vi "BioFeedback21(v_0.2).vi"() -> ()   [LabVIEW 2016]
doc: "Use this template to build a producer/consumer design pattern. Use this template when you need to execute a process, such as data analysis, when a data source, such as a triggered acquisition, produces data at an uneven rate and you need to execute the process when the data becomes available."
uses:
  customSubVIs/8ChanWfmArray.ctl
  <vilib>/Utility/file.llb/Write Delimited Spreadsheet (string).vi
panel:
  in  "MVC Delay (s)":dbl=1.0
  out "trial last time":timestamp
  out "mvc last time":timestamp
  in  "Display Width for MVC (s)":dbl(slide) scale=0.1..10.0
  in  "Display Width for Current Trial":dbl(slide) scale=0.1..10.0
  out "Current Trial (Filtered)":waveform(dbl)(graph)
  out "Current MVC (Filtered)":waveform(dbl)(graph)
  in  "enableSave":bool caption="No Save      Save"
  in  "barOrGraph":bool=TRUE caption="Graph (under construction)       Bar"
  in  "Trial comment":string
  out "Collecting Data":bool
  in  "Display Min":dbl
  in  "Display Max":dbl=100.0
  in  "log filepath":path
  out "TrialStartTime":timestamp
  in  "Trial Duration (s)":dbl=3.0
  out "Trial Number":dbl
  in  "Session Name":string="Test"
  out "loopTime":dbl=30.0 caption="Upper Cut-Off"
  in  "trial display data":path
  out "Disp Data":cluster{"queue out":refnum<queue>, dbl, dbl}[](array[cluster])
  in  "Target Percentage":dbl=10.0
  out "Current Activation":dbl
  out "DisplayBarActivation":dbl(slide) caption="Percent Activation" max=1.0 scale=0.0..100.0
  in  "EMG Channel To Display":dbl=1.0
  out "MVC Data":cluster{"queue out":refnum<queue>, dbl, dbl}[](array[cluster])
  out "Trial Name":string="Test"
  in  "Data Directory":path=path "C:/Users/Tinggroup/Desktop/EMG Biofeedback System/LabviewFiles/Data"
  out "GetMaxStartTime":timestamp
  in  "MVC Number":dbl=1.0
  in  "MVC Duration (s)":dbl=3.0
  in  "Frames Per Second":dbl=30.0 caption="Upper Cut-Off"
  in  "EMG Input Device\nProduct Type":string="USB-6009"
  out "raw data":dynamicdata(graph)
  out "dispSize":dbl=20.0 caption="Lower Cut-Off"
  out "mvcSize":dbl=300.0 caption="Upper Cut-Off"
  in  "MVC Window Size (s)":dbl=0.5
  in  "Display Window Size (s)":dbl=0.5
  in  "MVC Raw Path":path
  in  "trial raw data":path
  in  "trial filtered data":path
  in  "MVC Filtered Path":path
  in  "Sample rate (Hz)":dbl=1000.0 caption="Upper Cut-Off"
  out "fps":dbl=20.0 caption="Lower Cut-Off"
  out "rate":dbl=300.0 caption="Upper Cut-Off"
  in  "Set Parameters":bool
  out "lower":dbl=20.0 caption="Lower Cut-Off"
  out "upper":dbl=300.0 caption="Upper Cut-Off"
  in  "Lower Cut-Off":dbl=20.0
  in  "Upper Cut-Off":dbl=500.0
  in  "Mark":bool
  in  "End Trial":bool
  in  "Get MVC":bool
  in  "StartTrial":bool
  out "State":T1(ring)
  out "FilteredAndRectified":waveform(dbl)[](graph) caption="Filtered and Rectified"
  in  "stop":bool
  # "Filtering"
  # "Add trial name\nBEFORE beginning trial"
  # "Display Settings"
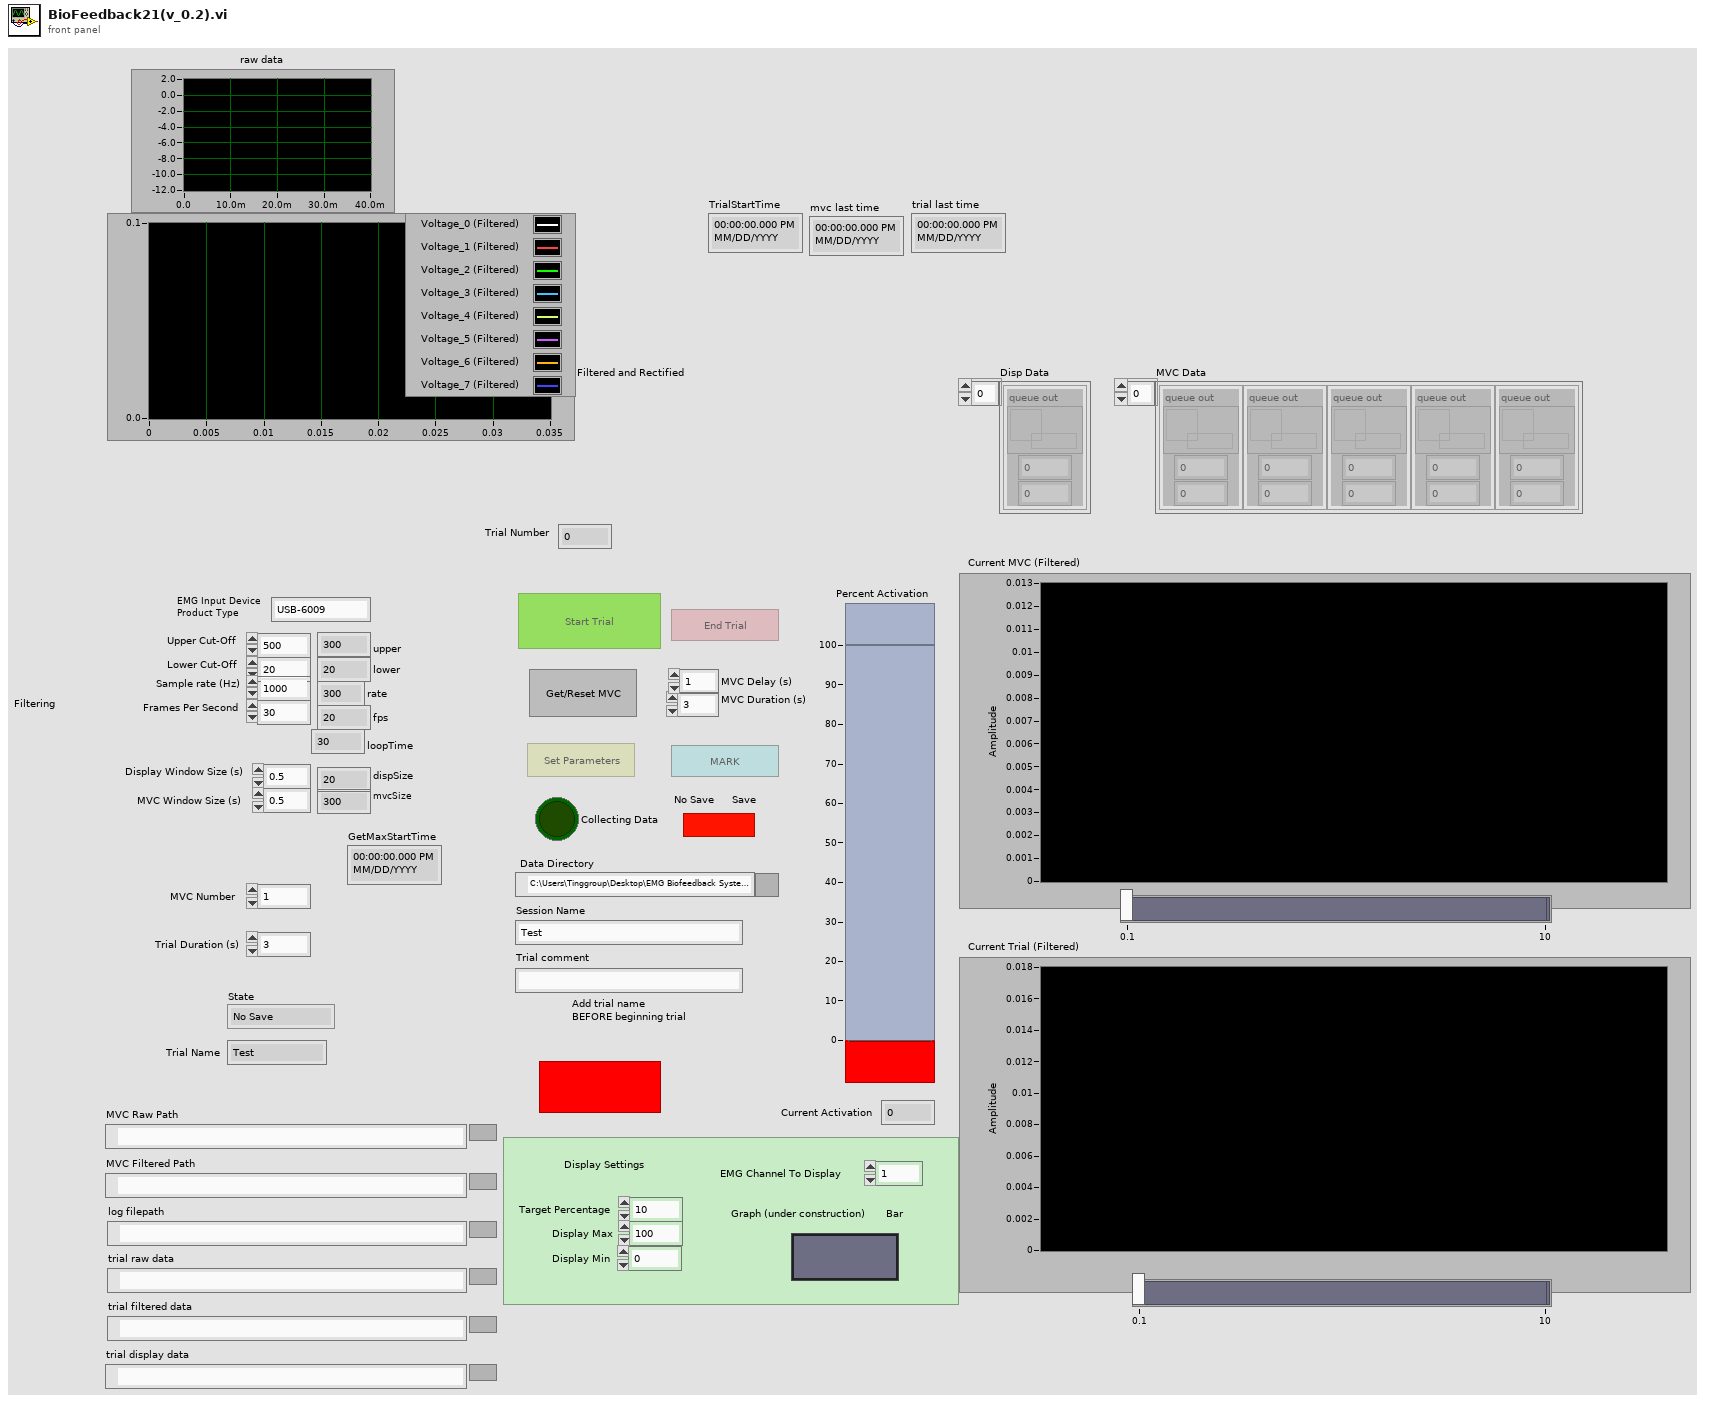
[diagram p1: front panel]
types:
  T1 = enum16{"No Save", "Acquiring Max", "Trial In Progress"}
  T2 = enum8{"Enabled", "Disabled", "Disabled and Grayed Out"}
  T3 = typedef "8ChanWfmArray.ctl" = waveform(dbl)[]
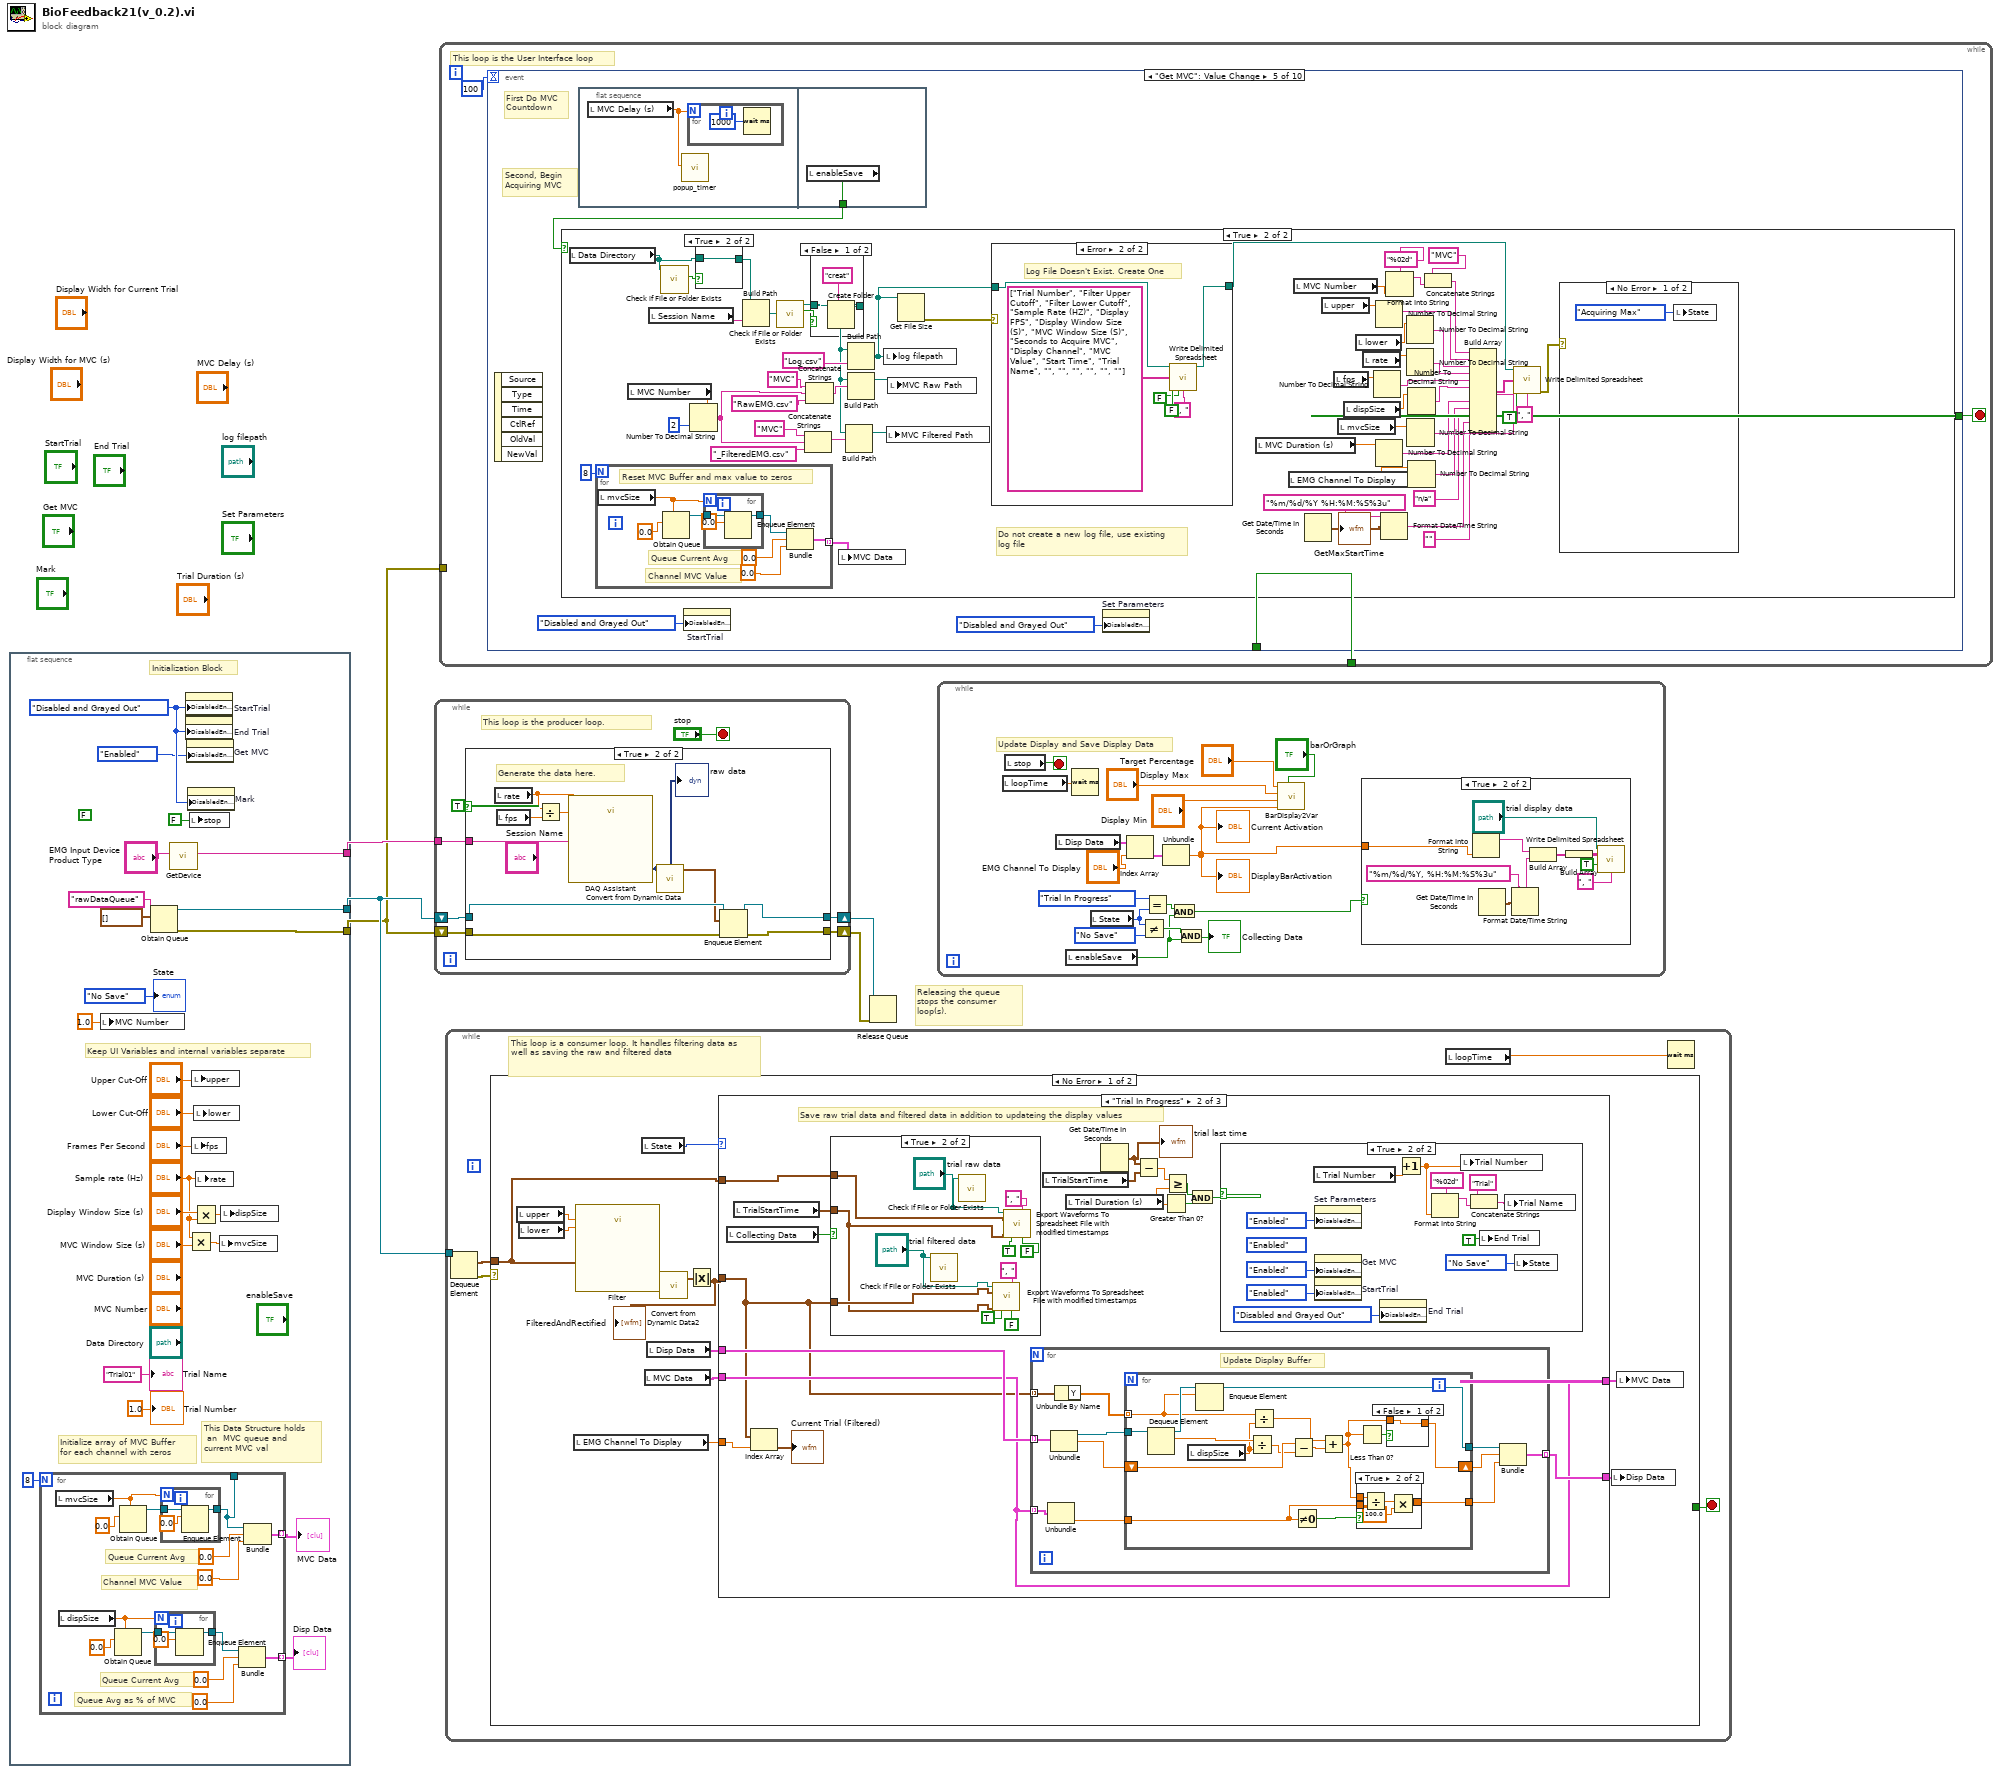
[diagram p0: block diagram]
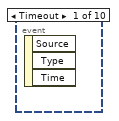
[diagram p3: hidden frame]
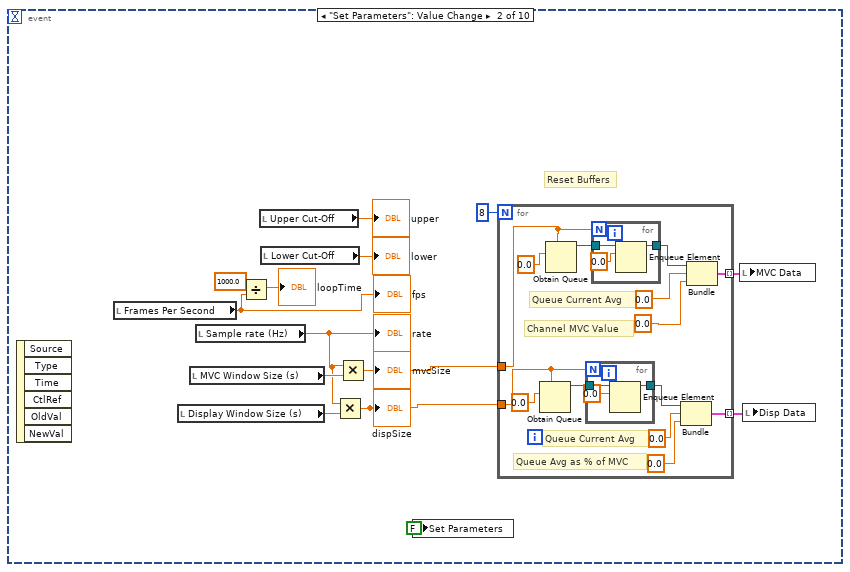
[diagram p4: hidden frame]
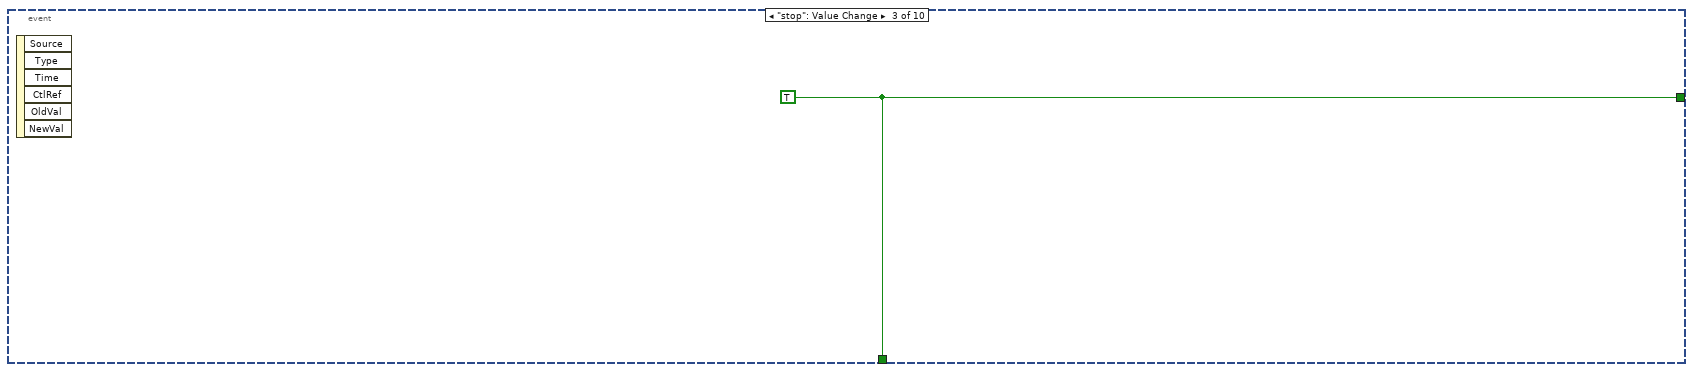
[diagram p5: hidden frame]
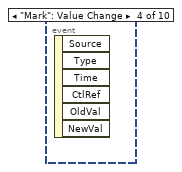
[diagram p6: hidden frame]
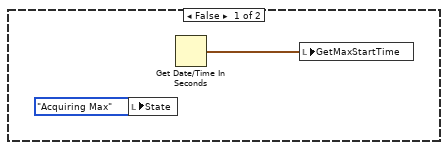
[diagram p7: hidden frame]
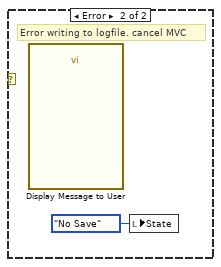
[diagram p8: hidden frame]
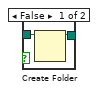
[diagram p11: hidden frame]
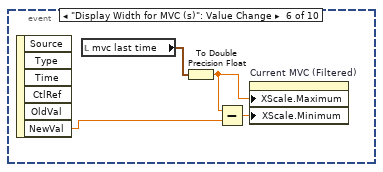
[diagram p12: hidden frame]
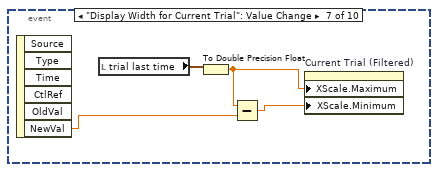
[diagram p13: hidden frame]
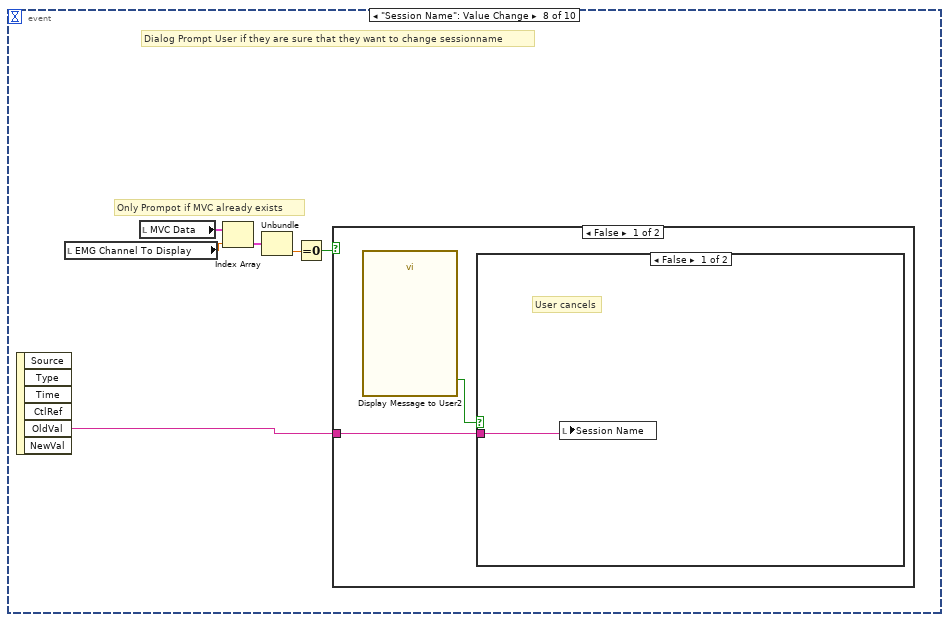
[diagram p14: hidden frame]
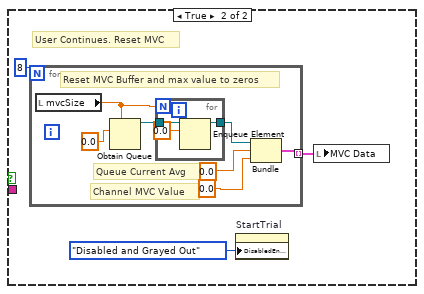
[diagram p15: hidden frame]
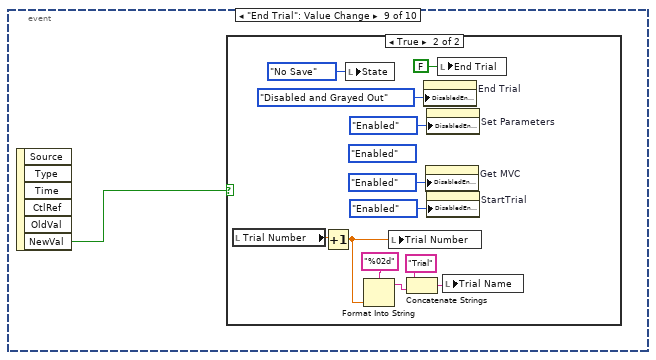
[diagram p17: hidden frame]
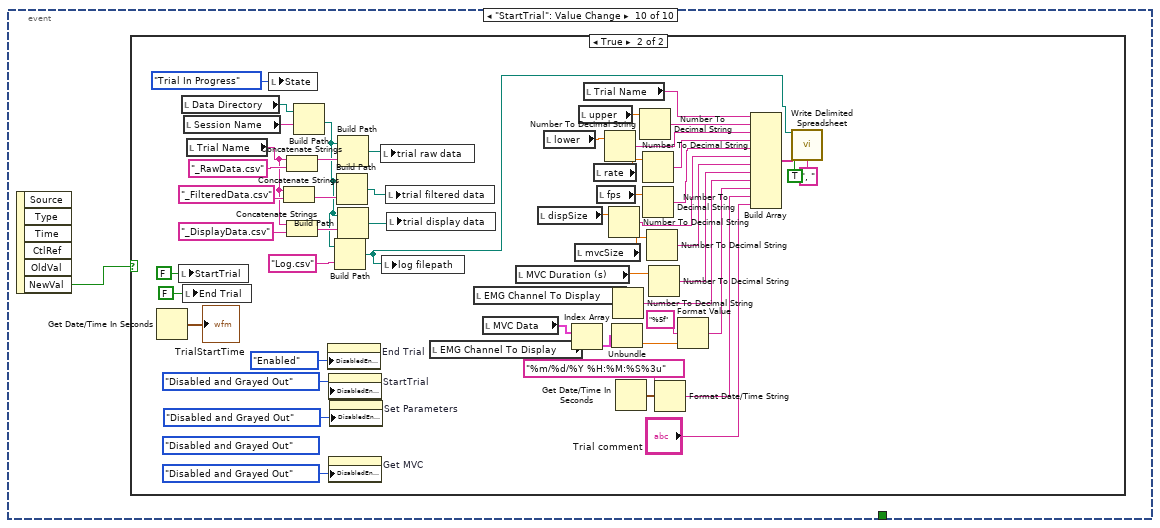
[diagram p19: hidden frame]
diagram:
  # "Releasing the queue stops the consumer loop(s)."
  n1 = flat-sequence {
    tunnel: [w20] -> w3
    tunnel: [w19] -> w2
    tunnel: [w22] -> w4
    frame #0 {
      (unwired) FALSE ("Visible")
      w27 = T2."Disabled and Grayed Out" ("Disabled")
      # "Keep UI Variables and internal variables separate"
      # "This Data Structure holds\n an  MVC queue and \ncurrent MVC val"
      # "Initialize array of MVC Buffer \nfor each channel with zeros"
      # "Initialization Block"
      n2 = for {
        N: 8 -> [_]
        tunnel: [w40] -> w12 mode=indexing
        tunnel: [w37] -> _
        tunnel: [w30] -> w11 mode=indexing
        # "Queue Avg as % of MVC"
        # "Queue Current Avg"
        # "Channel MVC Value"
        # "Queue Current Avg"
        n3 = local read "mvcSize"() -> (w41:dbl)
        n4 = local read "dispSize"() -> (w34:dbl)
        n5 = Obtain Queue(max queue size (-1, unlimited)=w34, element data type=0.0) -> (queue out=w31:refnum<queue>)  [unwired: 3 in, 2 out]
        n6 = Obtain Queue(max queue size (-1, unlimited)=w41, element data type=0.0) -> (queue out=w42:refnum<queue>)  [unwired: 3 in, 2 out]
        n7 = for {
          N: w34 -> [_]
          tunnel: w31 -> [w46]
          tunnel: [w44] -> w32
          n8 = Enqueue Element(queue=w46, element=0.0) -> (queue out=w44:refnum<queue>)  [unwired: 2 in, 2 out]
        }
        n9 = for {
          N: w41 -> [_]
          tunnel: w42 -> [w49]
          tunnel: [w47] -> w37
          n10 = Enqueue Element(queue=w49, element=0.0) -> (queue out=w47:refnum<queue>)  [unwired: 2 in, 2 out]
        }
        n11 = Bundle("queue out"=w32, 0.0, 0.0) -> (w30:cluster{"queue out":refnum<queue>, dbl, dbl})  [unwired: 1 in]
        n12 = Bundle("queue out"=w37, 0.0, 0.0) -> (w40:cluster{"queue out":refnum<queue>, dbl, dbl})  [unwired: 1 in]
      }
      "MVC Data" <- w12
      "Disp Data" <- w11
      n13 = local write "MVC Number"(1.0 ("MVC Number")) -> ()
      n14 = Obtain Queue(name (unnamed)="rawDataQueue", element data type=T3 [] ("initialized array")) -> (queue out=w20:refnum<queue>, error out=w19:errorcluster)  [unwired: 3 in, 1 out]
      n15 = call "GetDevice.vi"("EMG Input Device\nProduct Type"="EMG Input Device\nProduct Type") -> ("DAQmx Device Name"=w22:tag)  [unwired: 10 in]
      n16 = property on="StartTrial" class="Bool (strict)"("DisabledEnum"=w27) -> ()  [unwired: 2 in, 2 out]
      n17 = property on="End Trial" class="Bool (strict)"("DisabledEnum"=w27) -> ()  [unwired: 2 in, 2 out]
      n18 = property on="Get MVC" class="Bool"("DisabledEnum"=T2."Enabled" ("Disabled")) -> ()  [unwired: 2 in, 2 out]
      n19 = property on="Mark" class="Bool"("DisabledEnum"=w27) -> ()  [unwired: 2 in, 2 out]
      n20 = Multiply(x="Sample rate (Hz)", y="MVC Window Size (s)") -> (x*y=w14:dbl)
      n21 = local write "stop"(FALSE ("stop")) -> ()
      n22 = local write "upper"("Upper Cut-Off") -> ()
      n23 = local write "fps"("Frames Per Second") -> ()
      n24 = Multiply(x="Display Window Size (s)", y="Sample rate (Hz)") -> (x*y=w17:dbl)
      n25 = local write "lower"("Lower Cut-Off") -> ()
      n26 = local write "rate"("Sample rate (Hz)") -> ()
      n27 = local write "mvcSize"(w14) -> ()
      n28 = local write "dispSize"(w17) -> ()
      "Trial Name" <- "Trial01" ("Trial Name")
      "State" <- T1."No Save" ("State")
      "Trial Number" <- 1.0 ("Trial Number")
    }
  }
  n29 = while {
    shift-right: [w52] -> w1
    shift-left: w2 -> [w53]
    shift-right: [w54] -> w5
    shift-left: w3 -> [w55]
    tunnel: w4 -> [w50]
    stop <- "stop" stop-if-true
    # "This loop is the producer loop."
    n30 = case shown="True" TRUE ("Case Constant\n(See Context Help)") {
      tunnel: w55 -> [w58 w68]
      tunnel: [w58 w67] -> w54
      tunnel: w53 -> [w57 w66]
      tunnel: [w57 w65] -> w52
      tunnel: w50 -> [_ w60]
      frame False {
      }
      frame True {
        # "Generate the data here."
        n31 = local read "rate"() -> (w63:dbl)
        n32 = local read "fps"() -> (w64:dbl)
        n33 = Divide(x=w63, y=w64) -> (x/y=w62:dbl)
        n34 = call "DAQ Assistant"("rate"=w63, "number of samples"=w62, "device name"=w60) -> ("data"=w61:dynamicdata)  [unwired: 13 in, 3 out]
        "raw data" <- w61
        n35 = call "Convert from Dynamic Data"("Dynamic Data Type"=w61) -> ("Array of Waveform"=w59:waveform(dbl)[])  [unwired: 3 in]
        n36 = Enqueue Element(queue=w68, element=w59, error in (no error)=w66) -> (queue out=w67:refnum<queue>, error out=w65:errorcluster)  [unwired: 1 in, 1 out]
      }
    }
  }
  n37 = while {
    tunnel: [w71] -> _
    tunnel: w2 -> [_]
    stop <- w69 stop-if-true
    # "This loop is the User Interface loop"
    n38 = event shown="[4] \"Get MVC\": Value Change" {
      selector: _ -> [_ _ _ _ _ _ _ _ _ _]
      dyn-events: _ -> [_ _ _ _ _ _ _ _ _ _]
      timeout: u32 100 ("milliseconds to wait") -> [_ _ _ _ _ _ _ _ _ _]
      tunnel: [_ _ w106 _ _ _ _ _ _ _] -> w69
      tunnel: [_ _ w106 _ _ _ _ _ _ _] -> w71
      event Timeout {
        n39 = event-data() -> ()  [unwired: 1 in, 3 out]
      }
      event "Set Parameters": Value Change {
        # "Reset Buffers"
        n40 = event-data() -> ()  [unwired: 1 in, 6 out]
        n41 = local read "Frames Per Second"() -> (w73:dbl)
        "fps" <- w73
        n42 = local read "Display Window Size (s)"() -> (w83:dbl)
        n43 = local read "MVC Window Size (s)"() -> (w84:dbl)
        n44 = local read "Sample rate (Hz)"() -> (w81:dbl)
        "rate" <- w81
        n45 = Divide(x=1000.0, y=w73) -> (x/y=→"loopTime":dbl)
        n46 = local read "Upper Cut-Off"() -> (→"upper":dbl)
        n47 = local read "Lower Cut-Off"() -> (→"lower":dbl)
        n48 = Multiply(x=w81, y=w83) -> (x*y=w79:dbl)
        "dispSize" <- w79
        n49 = Multiply(x=w81, y=w84) -> (x*y=w80:dbl)
        "mvcSize" <- w80
        n50 = local write "Set Parameters"(FALSE ("Set Parameters")) -> ()
        n51 = for {
          N: 8 -> [_]
          tunnel: [w97] -> w77 mode=indexing
          tunnel: [w88] -> w78 mode=indexing
          tunnel: w80 -> [w87]
          tunnel: w79 -> [w86]
          # "Queue Avg as % of MVC"
          # "Queue Current Avg"
          # "Channel MVC Value"
          # "Queue Current Avg"
          n52 = Obtain Queue(max queue size (-1, unlimited)=w86, element data type=0.0) -> (queue out=w89:refnum<queue>)  [unwired: 3 in, 2 out]
          n53 = Obtain Queue(max queue size (-1, unlimited)=w87, element data type=0.0) -> (queue out=w98:refnum<queue>)  [unwired: 3 in, 2 out]
          n54 = for {
            N: w86 -> [_]
            tunnel: w89 -> [w102]
            tunnel: [w100] -> w90
            n55 = Enqueue Element(queue=w102, element=0.0) -> (queue out=w100:refnum<queue>)  [unwired: 2 in, 2 out]
          }
          n56 = for {
            N: w87 -> [_]
            tunnel: w98 -> [w105]
            tunnel: [w103] -> w94
            n57 = Enqueue Element(queue=w105, element=0.0) -> (queue out=w103:refnum<queue>)  [unwired: 2 in, 2 out]
          }
          n58 = Bundle("queue out"=w90, 0.0, 0.0) -> (w88:cluster{"queue out":refnum<queue>, dbl, dbl})  [unwired: 1 in]
          n59 = Bundle("queue out"=w94, 0.0, 0.0) -> (w97:cluster{"queue out":refnum<queue>, dbl, dbl})  [unwired: 1 in]
        }
        n60 = local write "MVC Data"(w77) -> ()
        n61 = local write "Disp Data"(w78) -> ()
      }
      event "stop": Value Change {
        w106 = TRUE
        n62 = event-data() -> ()  [unwired: 1 in, 6 out]
      }
      event "Mark": Value Change {
        n63 = event-data() -> ()  [unwired: 1 in, 6 out]
      }
      event "Get MVC": Value Change {
        # "Second, Begin \nAcquiring MVC"
        # "First Do MVC\nCountdown"
        n64 = event-data() -> ()  [unwired: 1 in, 6 out]
        n65 = case shown="True" w107 {
          frame False {
            n66 = local write "State"(T1."Acquiring Max" ("State")) -> ()
            n67 = Get Date/Time In Seconds() -> (seconds since 1Jan1904=w113:timestamp)
            n68 = local write "GetMaxStartTime"(w113) -> ()
          }
          frame True {
            # "Do not create a new log file, use existing \nlog file"
            n69 = local read "Data Directory"() -> (w122:path)
            n70 = for {
              N: 8 -> [_]
              tunnel: [w172] -> w119 mode=indexing
              # "Channel MVC Value"
              # "Queue Current Avg"
              # "Reset MVC Buffer and max value to zeros"
              n71 = local read "mvcSize"() -> (w175:dbl)
              n72 = Obtain Queue(max queue size (-1, unlimited)=w175, element data type=0.0) -> (queue out=w174:refnum<queue>)  [unwired: 3 in, 2 out]
              n73 = for {
                N: w175 -> [_]
                tunnel: w174 -> [w181]
                tunnel: [w179] -> w176
                n74 = Enqueue Element(queue=w181, element=0.0) -> (queue out=w179:refnum<queue>)  [unwired: 2 in, 2 out]
              }
              n75 = Bundle("queue out"=w176, 0.0, 0.0) -> (w172:cluster{"queue out":refnum<queue>, dbl, dbl})  [unwired: 1 in]
            }
            n76 = local read "MVC Number"() -> (w163:dbl)
            n77 = local read "Session Name"() -> (w162:string)
            n78 = call <vilib>:"Check if File or Folder Exists.vi"("path"=w122) -> ("file or folder exists?"=w123:bool)  [unwired: 8 in, 2 out]
            n79 = Number To Decimal String(number=w163, width (-)=i16 2) -> (decimal integer string=w144:string)
            n80 = case shown="True" w123 {
              tunnel: [w194 w195] -> w158
              tunnel: w122 -> [w193 w195]
              frame False {
                n81 = Create Folder(path (use dialog)=w193) -> (created path=w194:path)  [unwired: 2 in, 2 out]
              }
              frame True {
              }
            }
            n82 = Build Path(base path=w158, name or relative path=w162) -> (appended path=w161:path)
            n83 = call <vilib>:"Check if File or Folder Exists.vi"("path"=w161) -> ("file or folder exists?"=w160:bool, "dup path"=w159:path)  [unwired: 8 in, 1 out]
            n84 = Concatenate Strings("MVC" ("string"), w144, "_FilteredEMG.csv" ("string")) -> (w168:string)
            n85 = Concatenate Strings("MVC" ("string"), w144, "RawEMG.csv" ("string")) -> (w167:string)
            n86 = case shown="False" w160 {
              tunnel: w159 -> [w191 w192]
              tunnel: [w190 w192] -> w155
              frame False {
                n87 = Create Folder(prompt (Create Folder)="creat", path (use dialog)=w191) -> (created path=w190:path)  [unwired: 1 in, 2 out]
              }
              frame True {
              }
            }
            n88 = local write "MVC Data"(w119) -> ()
            n89 = Build Path(base path=w155, name or relative path=w168) -> (appended path=w120:path)
            n90 = Build Path(base path=w155, name or relative path="Log.csv" ("string")) -> (appended path=w116:path)
            n91 = Build Path(base path=w155, name or relative path=w167) -> (appended path=w121:path)
            n92 = local write "log filepath"(w116) -> ()
            n93 = local write "MVC Filtered Path"(w120) -> ()
            n94 = local write "MVC Raw Path"(w121) -> ()
            n95 = Get File Size(file=w116) -> (0:w115:errorcluster)  [unwired: 1 in, 2 out]
            n96 = case shown="Error" w115 {
              tunnel: [w182 w184] -> w135
              tunnel: w116 -> [w182 w183]
              frame No Error {
              }
              frame Error {
                # "Log File Doesn't Exist. Create One"
                n97 = call-poly <vilib>:"Write Delimited Spreadsheet.vi"("file path (dialog if empty)"=w183, "1D data"=string[] ["Trial Number", "Filter Upper Cutoff", "Filter Lower Cutoff", "Sample Rate (HZ)", "Display FPS", "Display Window Size (S)", "MVC Window Size (S)", "Seconds to Acquire MVC", "Display Channel", "MVC Value", "Start Time", "Trial Name", "", "", "", "", "", ""], "append to file? (new file:F)"=FALSE, "transpose? (no:F)"=FALSE, "delimiter (\\t)"=", " ("delimiter (\\t)")) -> ("new file path (Not A Path if cancelled)"=w184:path)  [unwired: 9 in, 1 out]
              }
            }
            n98 = local read "MVC Duration (s)"() -> (w149:dbl)
            n99 = local read "EMG Channel To Display"() -> (w148:dbl)
            n100 = local read "MVC Number"() -> (w131:dbl)
            n101 = Get Date/Time In Seconds() -> (seconds since 1Jan1904=w127:timestamp)
            "GetMaxStartTime" <- w127
            n102 = local read "upper"() -> (w154:dbl)
            n103 = local read "fps"() -> (w151:dbl)
            n104 = local read "mvcSize"() -> (w150:dbl)
            n105 = local read "dispSize"() -> (w145:dbl)
            n106 = local read "lower"() -> (w153:dbl)
            n107 = local read "rate"() -> (w152:dbl)
            n108 = Number To Decimal String(number=w151) -> (decimal integer string=w141:string)  [unwired: 1 in]
            n109 = Number To Decimal String(number=w154) -> (decimal integer string=w129:string)  [unwired: 1 in]
            n110 = Number To Decimal String(number=w149) -> (decimal integer string=w138:string)  [unwired: 1 in]
            n111 = Format Date/Time String(time format string (%c)="%m/%d/%Y %H:%M:%S%3u", seconds (now)=w127) -> (date/time string=w125:string)  [unwired: 1 in]
            n112 = Format Into String(format string="%02d", w131) -> (resulting string=w134:string)  [unwired: 2 in, 1 out]
            n113 = Number To Decimal String(number=w153) -> (decimal integer string=w143:string)  [unwired: 1 in]
            n114 = Number To Decimal String(number=w152) -> (decimal integer string=w142:string)  [unwired: 1 in]
            n115 = Number To Decimal String(number=w150) -> (decimal integer string=w139:string)  [unwired: 1 in]
            n116 = Number To Decimal String(number=w145) -> (decimal integer string=w140:string)  [unwired: 1 in]
            n117 = Number To Decimal String(number=w148) -> (decimal integer string=w137:string)  [unwired: 1 in]
            n118 = Concatenate Strings("MVC" ("string"), w134) -> (w130:string)
            n119 = Build Array(w130, w129, w143, w142, w141, w140, w139, w138, w137, "n/a", w125, "" ("element")) -> (w147:string[])
            n120 = call-poly <vilib>:"Write Delimited Spreadsheet.vi"("file path (dialog if empty)"=w135, "1D data"=w147, "append to file? (new file:F)"=TRUE, "delimiter (\\t)"=", " ("delimiter (\\t)")) -> ("error out"=w117:errorcluster)  [unwired: 10 in, 1 out]
            n121 = case shown="No Error" w117 {
              frame No Error {
                n122 = local write "State"(T1."Acquiring Max" ("State")) -> ()
              }
              frame Error {
                # "Error writing to logfile. cancel MVC"
                n123 = call "Display Message to User"() -> ()  [unwired: 10 in, 2 out]
                n124 = local write "State"(T1."No Save" ("State")) -> ()
              }
            }
          }
        }
        n125 = flat-sequence {
          tunnel: [w112] -> w107
          frame #0 {
            n126 = local read "MVC Delay (s)"() -> (w110:dbl)
            n127 = call "popup_timer.vi"("Seconds"=w110) -> ()  [unwired: 9 in, 1 out]
            n128 = for {
              N: w110 -> [_]
              n129 = Wait (ms)(milliseconds to wait=u32 1000) -> ()  [unwired: 1 out]
            }
          }
          frame #1 {
            n130 = local read "enableSave"() -> (w112:bool)
          }
        }
        n131 = property on="StartTrial" class="Bool (strict)"("DisabledEnum"=T2."Disabled and Grayed Out" ("Disabled")) -> ()  [unwired: 2 in, 2 out]
        n132 = property on="Set Parameters" class="Bool (strict)"("DisabledEnum"=T2."Disabled and Grayed Out" ("Disabled")) -> ()  [unwired: 2 in, 2 out]
      }
      event "Display Width for MVC (s)": Value Change {
        n133 = event-data() -> ("NewVal"=w199:dbl)  [unwired: 1 in, 5 out]
        n134 = local read "mvc last time"() -> (w196:timestamp)
        n135 = To Double Precision Float(number=w196) -> (double precision float=w197:dbl)
        n136 = Subtract(x=w197, y=w199) -> (x-y=w198:dbl)
        n137 = property on="Current MVC (Filtered)" class="WFChart (strict)"("XScale.Maximum"=w197, "XScale.Minimum"=w198) -> ()  [unwired: 2 in, 2 out]
      }
      event "Display Width for Current Trial": Value Change {
        n138 = event-data() -> ("NewVal"=w202:dbl)  [unwired: 1 in, 5 out]
        n139 = local read "trial last time"() -> (w203:timestamp)
        n140 = To Double Precision Float(number=w203) -> (double precision float=w201:dbl)
        n141 = Subtract(x=w201, y=w202) -> (x-y=w200:dbl)
        n142 = property on="Current Trial (Filtered)" class="WFChart (strict)"("XScale.Maximum"=w201, "XScale.Minimum"=w200) -> ()  [unwired: 2 in, 2 out]
      }
      event "Session Name": Value Change {
        # "Only Prompot if MVC already exists"
        # "Dialog Prompt User if they are sure that they want to change sessionname"
        n143 = event-data() -> ("OldVal"=w204:string)  [unwired: 1 in, 5 out]
        n144 = local read "EMG Channel To Display"() -> (w208:dbl)
        n145 = local read "MVC Data"() -> (w209:cluster{"queue out":refnum<queue>, dbl, dbl}[])
        n146 = Index Array(array=w209, index=w208) -> (element=w207:cluster{"queue out":refnum<queue>, dbl, dbl})
        n147 = Unbundle(w207) -> (w206:dbl)  [unwired: 2 out]
        n148 = Equal To 0?(x=w206) -> (x = 0?=w205:bool)
        n149 = case shown="False" w205 {
          tunnel: w204 -> [w210 _]
          frame False {
            n150 = call "Display Message to User2"() -> ("Change"=w211:bool)  [unwired: 10 in, 1 out]
            n151 = case shown="False" w211 {
              tunnel: w210 -> [w212 _]
              frame False {
                # "User cancels"
                n152 = local write "Session Name"(w212) -> ()
              }
              frame True {
                # "User Continues. Reset MVC"
                n153 = for {
                  N: 8 -> [_]
                  tunnel: [w216] -> w215 mode=indexing
                  # "Channel MVC Value"
                  # "Queue Current Avg"
                  # "Reset MVC Buffer and max value to zeros"
                  n154 = local read "mvcSize"() -> (w219:dbl)
                  n155 = Obtain Queue(max queue size (-1, unlimited)=w219, element data type=0.0) -> (queue out=w218:refnum<queue>)  [unwired: 3 in, 2 out]
                  n156 = for {
                    N: w219 -> [_]
                    tunnel: w218 -> [w225]
                    tunnel: [w223] -> w220
                    n157 = Enqueue Element(queue=w225, element=0.0) -> (queue out=w223:refnum<queue>)  [unwired: 2 in, 2 out]
                  }
                  n158 = Bundle("queue out"=w220, 0.0, 0.0) -> (w216:cluster{"queue out":refnum<queue>, dbl, dbl})  [unwired: 1 in]
                }
                n159 = property on="StartTrial" class="Bool (strict)"("DisabledEnum"=T2."Disabled and Grayed Out" ("Disabled")) -> ()  [unwired: 2 in, 2 out]
                n160 = local write "MVC Data"(w215) -> ()
              }
            }
          }
          frame True {
          }
        }
      }
      event "End Trial": Value Change {
        n161 = event-data() -> ("NewVal"=w226:bool)  [unwired: 1 in, 5 out]
        n162 = case shown="True" w226 {
          frame False {
          }
          frame True {
            (unwired) T2."Enabled" ("Disabled")
            n163 = local read "Trial Number"() -> (w231:dbl)
            n164 = Increment(x=w231) -> (x+1=w227:dbl)
            n165 = local write "State"(T1."No Save" ("State")) -> ()
            n166 = Format Into String(format string="%02d", w227) -> (resulting string=w230:string)  [unwired: 2 in, 1 out]
            n167 = local write "Trial Number"(w227) -> ()
            n168 = Concatenate Strings("Trial" ("string"), w230) -> (w232:string)
            n169 = property on="End Trial" class="Bool (strict)"("DisabledEnum"=T2."Disabled and Grayed Out" ("Disabled")) -> ()  [unwired: 2 in, 2 out]
            n170 = property on="Get MVC" class="Bool"("DisabledEnum"=T2."Enabled" ("Disabled")) -> ()  [unwired: 2 in, 2 out]
            n171 = property on="Set Parameters" class="Bool (strict)"("DisabledEnum"=T2."Enabled" ("Disabled")) -> ()  [unwired: 2 in, 2 out]
            n172 = property on="StartTrial" class="Bool (strict)"("DisabledEnum"=T2."Enabled" ("Disabled")) -> ()  [unwired: 2 in, 2 out]
            n173 = local write "End Trial"(FALSE ("End Trial")) -> ()
            n174 = local write "Trial Name"(w232) -> ()
          }
        }
      }
      event "StartTrial": Value Change {
        n175 = event-data() -> ("NewVal"=w239:bool)  [unwired: 1 in, 5 out]
        n176 = case shown="True" w239 {
          frame False {
          }
          frame True {
            (unwired) T2."Disabled and Grayed Out" ("Disabled")
            n177 = Get Date/Time In Seconds() -> (seconds since 1Jan1904=→"TrialStartTime":timestamp)
            n178 = local write "StartTrial"(FALSE ("StartTrial")) -> ()
            n179 = local read "Data Directory"() -> (w284:path)
            n180 = local write "End Trial"(FALSE ("End Trial")) -> ()
            n181 = local read "Session Name"() -> (w283:string)
            n182 = local read "Trial Name"() -> (w267:string)
            n183 = local write "State"(T1."Trial In Progress" ("State")) -> ()
            n184 = Concatenate Strings(w267, "_FilteredData.csv" ("string")) -> (w288:string)
            n185 = Concatenate Strings(w267, "_RawData.csv" ("string")) -> (w286:string)
            n186 = Concatenate Strings(w267, "_DisplayData.csv" ("string")) -> (w290:string)
            n187 = Build Path(base path=w284, name or relative path=w283) -> (appended path=w266:path)
            n188 = property on="End Trial" class="Bool (strict)"("DisabledEnum"=T2."Enabled" ("Disabled")) -> ()  [unwired: 2 in, 2 out]
            n189 = property on="StartTrial" class="Bool (strict)"("DisabledEnum"=T2."Disabled and Grayed Out" ("Disabled")) -> ()  [unwired: 2 in, 2 out]
            n190 = property on="Get MVC" class="Bool"("DisabledEnum"=T2."Disabled and Grayed Out" ("Disabled")) -> ()  [unwired: 2 in, 2 out]
            n191 = property on="Set Parameters" class="Bool (strict)"("DisabledEnum"=T2."Disabled and Grayed Out" ("Disabled")) -> ()  [unwired: 2 in, 2 out]
            n192 = Build Path(base path=w266, name or relative path="Log.csv" ("string")) -> (appended path=w250:path)
            n193 = Build Path(base path=w266, name or relative path=w288) -> (appended path=w282:path)
            n194 = Build Path(base path=w266, name or relative path=w286) -> (appended path=w281:path)
            n195 = Build Path(base path=w266, name or relative path=w290) -> (appended path=w291:path)
            n196 = local write "trial raw data"(w281) -> ()
            n197 = local write "log filepath"(w250) -> ()
            n198 = local write "trial filtered data"(w282) -> ()
            n199 = local write "trial display data"(w291) -> ()
            n200 = local read "EMG Channel To Display"() -> (w246:dbl)
            n201 = local read "EMG Channel To Display"() -> (w276:dbl)
            n202 = local read "MVC Data"() -> (w247:cluster{"queue out":refnum<queue>, dbl, dbl}[])
            n203 = local read "MVC Duration (s)"() -> (w275:dbl)
            n204 = local read "dispSize"() -> (w273:dbl)
            n205 = local read "lower"() -> (w270:dbl)
            n206 = Index Array(array=w247, index=w246) -> (element=w245:cluster{"queue out":refnum<queue>, dbl, dbl})
            n207 = local read "mvcSize"() -> (w274:dbl)
            n208 = local read "upper"() -> (w269:dbl)
            n209 = local read "Trial Name"() -> (w263:string)
            n210 = local read "rate"() -> (w271:dbl)
            n211 = local read "fps"() -> (w272:dbl)
            n212 = Number To Decimal String(number=w270) -> (decimal integer string=w259:string)  [unwired: 1 in]
            n213 = Number To Decimal String(number=w273) -> (decimal integer string=w257:string)  [unwired: 1 in]
            n214 = Unbundle(w245) -> (w241:dbl)  [unwired: 2 out]
            n215 = Number To Decimal String(number=w276) -> (decimal integer string=w254:string)  [unwired: 1 in]
            n216 = Get Date/Time In Seconds() -> (seconds since 1Jan1904=w249:timestamp)
            n217 = Number To Decimal String(number=w269) -> (decimal integer string=w260:string)  [unwired: 1 in]
            n218 = Number To Decimal String(number=w271) -> (decimal integer string=w258:string)  [unwired: 1 in]
            n219 = Number To Decimal String(number=w272) -> (decimal integer string=w253:string)  [unwired: 1 in]
            n220 = Number To Decimal String(number=w274) -> (decimal integer string=w256:string)  [unwired: 1 in]
            n221 = Number To Decimal String(number=w275) -> (decimal integer string=w255:string)  [unwired: 1 in]
            n222 = Format Date/Time String(time format string (%c)="%m/%d/%Y %H:%M:%S%3u", seconds (now)=w249) -> (date/time string=w244:string)  [unwired: 1 in]
            n223 = Format Value(format string="%5f", value (0)=w241) -> (output string=w240:string)  [unwired: 1 in]
            n224 = Build Array(w263, w260, w259, w258, w253, w257, w256, w255, w254, w240, w244, "Trial comment") -> (w252:string[])
            n225 = call-poly <vilib>:"Write Delimited Spreadsheet.vi"("file path (dialog if empty)"=w250, "1D data"=w252, "append to file? (new file:F)"=TRUE, "delimiter (\\t)"=", " ("delimiter (\\t)")) -> ()  [unwired: 10 in, 2 out]
          }
        }
      }
    }
  }
  n226 = while {
    tunnel: w3 -> [w294]
    stop <- w295 stop-if-true
    # "This loop is a consumer loop. It handles filtering data as well as saving the raw and filtered data"
    n227 = Dequeue Element(queue=w294) -> (element=w296:T3, error out=w297:errorcluster)  [unwired: 2 in, 2 out]
    n228 = case shown="No Error" w297 {
      tunnel: w296 -> [w305 _]
      tunnel: [_ TRUE] -> w295
      frame No Error {
        n229 = local read "upper"() -> (w307:dbl)
        n230 = local read "lower"() -> (w306:dbl)
        n231 = local read "EMG Channel To Display"() -> (w298:dbl)
        n232 = call "Filter"("Lower Cut-Off"=w306, "Upper Cut-Off"=w307, "Signal"=w305) -> ("Filtered Signal"=w308:dynamicdata)  [unwired: 7 in, 1 out]
        n233 = local read "State"() -> (w299:T1)
        n234 = local read "MVC Data"() -> (w303:cluster{"queue out":refnum<queue>, dbl, dbl}[])
        n235 = local read "Disp Data"() -> (w302:cluster{"queue out":refnum<queue>, dbl, dbl}[])
        n236 = call "Convert from Dynamic Data2"("Dynamic Data Type"=w308) -> ("Array of Waveform"=w309:waveform(dbl)[])  [unwired: 3 in]
        n237 = Absolute Value(x=w309) -> (abs(x)=w304:waveform(dbl)[])
        "FilteredAndRectified" <- w304
        n238 = case shown="\"Trial In Progress\"" w299 {
          tunnel: w304 -> [w313 w351 w425]
          tunnel: w305 -> [_ w355 w430]
          tunnel: w303 -> [w310 w362 w433]
          tunnel: w302 -> [w312 w364 w432]
          tunnel: [w311 w363 w428] -> w300
          tunnel: [w310 w362 w429] -> w301
          tunnel: w298 -> [_ w352 w426]
          frame "No Save", Default {
            # "Update the display values, but do not save anything\n\nNote: MVC data is just referenced to calculate percent activation"
            n239 = for {
              tunnel: w312 -> [w318] mode=indexing
              tunnel: w313 -> [w323] mode=indexing
              tunnel: [w319] -> w311 mode=indexing
              tunnel: w310 -> [w316] mode=indexing
              # "Update Display Buffer"
              n240 = Unbundle(w316) -> (w315:dbl)  [unwired: 2 out]
              n241 = Unbundle(w318) -> ("queue out"=w324:refnum<queue>, w317:dbl)  [unwired: 1 out]
              n242 = Unbundle By Name(w323) -> ("Y"=w322:dbl[])
              n243 = for {
                tunnel: w324 -> [w334]
                tunnel: w322 -> [w330] mode=indexing
                shift-right: [w327] -> w321
                shift-left: w317 -> [w339]
                tunnel: [w329] -> w320
                tunnel: w315 -> [w332]
                tunnel: [w328] -> w314
                n244 = Dequeue Element(queue=w334) -> (queue out=w331:refnum<queue>, element=w340:dbl)  [unwired: 2 in, 2 out]
                n245 = local read "dispSize"() -> (w337:dbl)
                n246 = Enqueue Element(queue=w331, element=w330) -> (queue out=w329:refnum<queue>)  [unwired: 2 in, 2 out]
                n247 = Divide(x=w340, y=w337) -> (x/y=w338:dbl)
                n248 = Divide(x=w330, y=w337) -> (x/y=w335:dbl)
                n249 = Subtract(x=w339, y=w338) -> (x-y=w336:dbl)
                n250 = Not Equal To 0?(x=w332) -> (x != 0?=w333:bool)
                n251 = Add(x=w335, y=w336) -> (x+y=w325:dbl)
                n252 = Less Than 0?(x=w325) -> (x < 0?=w326:bool)
                n253 = case shown="True" w333 {
                  tunnel: w332 -> [_ w348]
                  tunnel: [0.0 w344] -> w328
                  tunnel: w325 -> [_ w347]
                  frame False {
                  }
                  frame True {
                    n254 = Divide(x=w347, y=w348) -> (x/y=w345:dbl)
                    n255 = Multiply(x=w345, y=100.0) -> (x*y=w344:dbl)
                  }
                }
                n256 = case shown="True" w326 {
                  tunnel: [w341 0.0] -> w327
                  tunnel: w325 -> [w341 _]
                  frame False {
                  }
                  frame True {
                  }
                }
              }
              n257 = Bundle("queue out"=w320, w321, w314) -> (w319:cluster{"queue out":refnum<queue>, dbl, dbl})  [unwired: 1 in]
            }
          }
          frame "Trial In Progress" {
            # "Save raw trial data and filtered data in addition to updateing the display values"
            n258 = local read "Collecting Data"() -> (w354:bool)
            n259 = local read "TrialStartTime"() -> (w353:timestamp)
            n260 = Index Array(array=w351, index=w352) -> (element=→"Current Trial (Filtered)":waveform(dbl))
            n261 = case shown="True" w354 {
              tunnel: w351 -> [_ w373]
              tunnel: w355 -> [_ w367]
              tunnel: w353 -> [_ w368]
              frame False {
              }
              frame True {
                n262 = call <vilib>:"Check if File or Folder Exists.vi"("path"="trial filtered data") -> ()  [unwired: 8 in, 3 out]
                n263 = call <vilib>:"Check if File or Folder Exists.vi"("path"="trial raw data") -> ()  [unwired: 8 in, 3 out]
                n264 = call "Export Waveforms To Spreadsheet File with modified timestamps.vi"("file path (dialog if empty)"="trial filtered data", "delimiter (Tab)"=", ", "waveforms"=w373, "trial start time"=w368, "append to file? (new file:F)"=TRUE, "header? (write header:T)"=FALSE) -> ()  [unwired: 8 in, 2 out]
                n265 = call "Export Waveforms To Spreadsheet File with modified timestamps.vi"("file path (dialog if empty)"="trial raw data", "delimiter (Tab)"=", ", "waveforms"=w367, "trial start time"=w368, "append to file? (new file:F)"=TRUE, "header? (write header:T)"=FALSE) -> ()  [unwired: 8 in, 2 out]
              }
            }
            n266 = for {
              tunnel: w364 -> [w392] mode=indexing
              tunnel: w351 -> [w397] mode=indexing
              tunnel: [w393] -> w363 mode=indexing
              tunnel: w362 -> [w390] mode=indexing
              # "Update Display Buffer"
              n267 = Unbundle(w390) -> (w389:dbl)  [unwired: 2 out]
              n268 = Unbundle(w392) -> ("queue out"=w398:refnum<queue>, w391:dbl)  [unwired: 1 out]
              n269 = Unbundle By Name(w397) -> ("Y"=w396:dbl[])
              n270 = for {
                tunnel: w398 -> [w408]
                tunnel: w396 -> [w404] mode=indexing
                shift-right: [w399] -> w395
                shift-left: w391 -> [w413]
                tunnel: [w403] -> w394
                tunnel: w389 -> [w406]
                tunnel: [w402] -> w388
                n271 = Dequeue Element(queue=w408) -> (queue out=w405:refnum<queue>, element=w414:dbl)  [unwired: 2 in, 2 out]
                n272 = local read "dispSize"() -> (w411:dbl)
                n273 = Enqueue Element(queue=w405, element=w404) -> (queue out=w403:refnum<queue>)  [unwired: 2 in, 2 out]
                n274 = Divide(x=w414, y=w411) -> (x/y=w412:dbl)
                n275 = Divide(x=w404, y=w411) -> (x/y=w409:dbl)
                n276 = Subtract(x=w413, y=w412) -> (x-y=w410:dbl)
                n277 = Not Equal To 0?(x=w406) -> (x != 0?=w407:bool)
                n278 = Add(x=w409, y=w410) -> (x+y=w400:dbl)
                n279 = case shown="True" w407 {
                  tunnel: w406 -> [_ w422]
                  tunnel: [0.0 w420] -> w402
                  tunnel: w400 -> [_ w421]
                  frame False {
                  }
                  frame True {
                    n280 = Divide(x=w421, y=w422) -> (x/y=w419:dbl)
                    n281 = Multiply(x=w419, y=100.0) -> (x*y=w420:dbl)
                  }
                }
                n282 = Less Than 0?(x=w400) -> (x < 0?=w401:bool)
                n283 = case shown="False" w401 {
                  tunnel: [w415 0.0] -> w399
                  tunnel: w400 -> [w415 _]
                  frame False {
                  }
                  frame True {
                  }
                }
              }
              n284 = Bundle("queue out"=w394, w395, w388) -> (w393:cluster{"queue out":refnum<queue>, dbl, dbl})  [unwired: 1 in]
            }
            n285 = local read "TrialStartTime"() -> (w360:timestamp)
            n286 = local read "Trial Duration (s)"() -> (w357:dbl)
            n287 = Get Date/Time In Seconds() -> (seconds since 1Jan1904=w349:timestamp)
            "trial last time" <- w349
            n288 = Subtract(x=w349, y=w360) -> (x-y=w361:dbl)
            n289 = Greater Than 0?(x=w357) -> (x > 0?=w358:bool)
            n290 = Greater Or Equal?(x=w361, y=w357) -> (x >= y?=w356:bool)
            n291 = And(x=w356, y=w358) -> (x .and. y?=w359:bool)
            n292 = case shown="True" w359 {
              frame False {
              }
              frame True {
                (unwired) T2."Enabled" ("Disabled")
                n293 = local read "Trial Number"() -> (w377:dbl)
                n294 = property on="Set Parameters" class="Bool (strict)"("DisabledEnum"=T2."Enabled" ("Disabled")) -> ()  [unwired: 2 in, 2 out]
                n295 = property on="Get MVC" class="Bool"("DisabledEnum"=T2."Enabled" ("Disabled")) -> ()  [unwired: 2 in, 2 out]
                n296 = property on="StartTrial" class="Bool (strict)"("DisabledEnum"=T2."Enabled" ("Disabled")) -> ()  [unwired: 2 in, 2 out]
                n297 = property on="End Trial" class="Bool (strict)"("DisabledEnum"=T2."Disabled and Grayed Out" ("Disabled")) -> ()  [unwired: 2 in, 2 out]
                n298 = Increment(x=w377) -> (x+1=w376:dbl)
                n299 = Format Into String(format string="%02d", w376) -> (resulting string=w382:string)  [unwired: 2 in, 1 out]
                n300 = local write "Trial Number"(w376) -> ()
                n301 = Concatenate Strings("Trial" ("string"), w382) -> (w386:string)
                n302 = local write "End Trial"(TRUE ("End Trial")) -> ()
                n303 = local write "Trial Name"(w386) -> ()
                n304 = local write "State"(T1."No Save" ("State")) -> ()
              }
            }
          }
          frame "Acquiring Max" {
            # "Automatically Stop Listening for Max after Acquire Max Time is elapsed"
            n305 = local read "GetMaxStartTime"() -> (w427:timestamp)
            n306 = local read "Collecting Data"() -> (w431:bool)
            n307 = Index Array(array=w425, index=w426) -> (element=→"Current MVC (Filtered)":waveform(dbl))
            n308 = case shown="True" w431 {
              tunnel: w430 -> [_ w440]
              tunnel: w425 -> [_ w446]
              tunnel: w427 -> [_ w441]
              frame False {
              }
              frame True {
                n309 = call "Export Waveforms To Spreadsheet File with modified timestamps.vi"("file path (dialog if empty)"="MVC Filtered Path", "delimiter (Tab)"=", ", "waveforms"=w446, "trial start time"=w441, "append to file? (new file:F)"=TRUE, "header? (write header:T)"=FALSE) -> ()  [unwired: 8 in, 2 out]
                n310 = call "Export Waveforms To Spreadsheet File with modified timestamps.vi"("file path (dialog if empty)"="MVC Raw Path", "delimiter (Tab)"=", ", "waveforms"=w440, "trial start time"=w441, "append to file? (new file:F)"=TRUE, "header? (write header:T)"=FALSE) -> ()  [unwired: 8 in, 2 out]
              }
            }
            n311 = local read "GetMaxStartTime"() -> (w437:timestamp)
            n312 = local read "MVC Duration (s)"() -> (w435:dbl)
            n313 = Get Date/Time In Seconds() -> (seconds since 1Jan1904=w423:timestamp)
            "mvc last time" <- w423
            n314 = for {
              tunnel: w425 -> [w470] mode=indexing
              tunnel: w433 -> [w468] mode=indexing
              tunnel: [w462] -> w429 mode=indexing
              tunnel: w432 -> [w460] mode=indexing
              tunnel: [w454] -> w428 mode=indexing
              # "For each channel, update Moving Average for each channel"
              n315 = Unbundle(w468) -> ("queue out"=w461:refnum<queue>, w467:dbl, w466:dbl)
              n316 = Unbundle By Name(w470) -> ("Y"=w469:dbl[])
              n317 = Unbundle(w460) -> ("queue out"=w456:refnum<queue>, w459:dbl)  [unwired: 1 out]
              n318 = for {
                tunnel: w469 -> [w479] mode=indexing
                shift-right: [w484] -> w464
                shift-left: w467 -> [w496]
                shift-right: [w488] -> w465
                shift-left: w461 -> [w487]
                shift-right: [w490] -> w463
                shift-left: w466 -> [w489]
                tunnel: w459 -> [w477]
                shift-right: [w472] -> w457
                shift-left: _ -> [_]
                shift-right: [w481] -> w458
                shift-left: w456 -> [w474]
                # "Update Max if necessary"
                # "Update MVC queue current avg and \nmax value for each data point"
                n319 = Dequeue Element(queue=w474) -> (queue out=w483:refnum<queue>, element=w482:dbl)  [unwired: 2 in, 2 out]
                n320 = local read "dispSize"() -> (w480:dbl)
                n321 = Dequeue Element(queue=w487) -> (queue out=w486:refnum<queue>, element=w485:dbl)  [unwired: 2 in, 2 out]
                n322 = Enqueue Element(queue=w483, element=w479) -> (queue out=w481:refnum<queue>)  [unwired: 2 in, 2 out]
                n323 = local read "mvcSize"() -> (w494:dbl)
                n324 = Divide(x=w482, y=w480) -> (x/y=w478:dbl)
                n325 = Enqueue Element(queue=w486, element=w479) -> (queue out=w488:refnum<queue>)  [unwired: 2 in, 2 out]
                n326 = Divide(x=w479, y=w480) -> (x/y=w476:dbl)
                n327 = Subtract(x=w477, y=w478) -> (x-y=w475:dbl)
                n328 = Divide(x=w485, y=w494) -> (x/y=w495:dbl)
                n329 = Divide(x=w479, y=w494) -> (x/y=w492:dbl)
                n330 = Add(x=w476, y=w475) -> (x+y=w471:dbl)
                n331 = Subtract(x=w496, y=w495) -> (x-y=w493:dbl)
                n332 = Add(x=w492, y=w493) -> (x+y=w484:dbl)
                n333 = Less Than 0?(x=w471) -> (x < 0?=w473:bool)
                n334 = Greater?(x=w484, y=w489) -> (0:w491:bool)
                n335 = case shown="True" w473 {
                  tunnel: [w497 0.0] -> w472
                  tunnel: w471 -> [w497 _]
                  frame False {
                  }
                  frame True {
                  }
                }
                n336 = case shown="False" w491 {
                  tunnel: w484 -> [_ w500]
                  tunnel: [w499 w500] -> w490
                  tunnel: w489 -> [w499 _]
                  frame False {
                  }
                  frame True {
                  }
                }
              }
              n337 = Bundle("queue out"=w458, w457, 0.0) -> (w454:cluster{"queue out":refnum<queue>, dbl, dbl})  [unwired: 1 in]
              n338 = Bundle("queue out"=w465, w464, w463) -> (w462:cluster{"queue out":refnum<queue>, dbl, dbl})  [unwired: 1 in]
            }
            n339 = Subtract(x=w423, y=w437) -> (x-y=w436:dbl)
            n340 = Greater Or Equal?(x=w436, y=w435) -> (x >= y?=w434:bool)
            n341 = case shown="True" w434 {
              frame False {
              }
              frame True {
                w450 = T2."Enabled" ("Disabled")
                n342 = local read "Collecting Data"() -> (w449:bool)
                n343 = property on="StartTrial" class="Bool (strict)"("DisabledEnum"=w450) -> ()  [unwired: 2 in, 2 out]
                n344 = property on="Set Parameters" class="Bool (strict)"("DisabledEnum"=w450) -> ()  [unwired: 2 in, 2 out]
                n345 = case shown="True" w449 {
                  frame False {
                  }
                  frame True {
                    n346 = local read "MVC Number"() -> (w453:dbl)
                    n347 = Increment(x=w453) -> (x+1=w452:dbl)
                    n348 = local write "MVC Number"(w452) -> ()
                  }
                }
                n349 = local write "State"(T1."No Save" ("State")) -> ()
              }
            }
          }
        }
        n350 = local write "Disp Data"(w300) -> ()
        n351 = local write "MVC Data"(w301) -> ()
      }
      frame Error {
        # "Return true for any case which should stop the loop."
      }
    }
    n352 = local read "loopTime"() -> (w293:dbl)
    n353 = Wait (ms)(milliseconds to wait=w293) -> ()  [unwired: 1 out]
  }
  n354 = Release Queue(queue=w5, error in (no error)=w1) -> ()  [unwired: 1 in, 3 out]
  n355 = while {
    stop <- w515 stop-if-true
    # "Update Display and Save Display Data"
    n356 = local read "loopTime"() -> (w514:dbl)
    n357 = local read "stop"() -> (w515:bool)
    n358 = local read "Disp Data"() -> (w518:cluster{"queue out":refnum<queue>, dbl, dbl}[])
    n359 = local read "enableSave"() -> (w505:bool)
    n360 = Wait (ms)(milliseconds to wait=w514) -> ()  [unwired: 1 out]
    n361 = local read "State"() -> (w506:T1)
    n362 = Index Array(array=w518, index="EMG Channel To Display") -> (element=w516:cluster{"queue out":refnum<queue>, dbl, dbl})
    n363 = Not Equal?(x=w506, y=T1."No Save" ("State")) -> (x != y?=w509:bool)
    n364 = Equal?(x=T1."Trial In Progress" ("State"), y=w506) -> (x = y?=w504:bool)
    n365 = Unbundle(w516) -> (w503:dbl)  [unwired: 2 out]
    "DisplayBarActivation" <- w503
    "Current Activation" <- w503
    n366 = And(x=w504, y=w505) -> (x .and. y?=w502:bool)
    n367 = And(x=w509, y=w505) -> (x .and. y?=→"Collecting Data":bool)
    n368 = call "BarDisplay2Var.vi"("barOrGraph"="barOrGraph", "Activation Percentage"=w503, "scale min"="Display Min", "scale max"="Display Max", "Target Percentage"="Target Percentage") -> ()  [unwired: 7 in]
    n369 = case shown="True" w502 {
      tunnel: w503 -> [_ w520]
      frame False {
      }
      frame True {
        n370 = Format Into String(w520) -> (resulting string=w525:string)  [unwired: 3 in, 1 out]
        n371 = Get Date/Time In Seconds() -> (seconds since 1Jan1904=w523:timestamp)
        n372 = Format Date/Time String(time format string (%c)="%m/%d/%Y, %H:%M:%S%3u", seconds (now)=w523) -> (date/time string=w524:string)  [unwired: 1 in]
        n373 = Build Array(w525, w524) -> (w526:string[])
        n374 = Build Array(w526) -> (w527:string[][])
        n375 = call-poly <vilib>:"Write Delimited Spreadsheet.vi"("file path (dialog if empty)"="trial display data", "2D data"=w527, "append to file? (new file:F)"=TRUE, "delimiter (\\t)"=", " ("delimiter (\\t)")) -> ()  [unwired: 10 in, 2 out]
      }
    }
  }
